vi "SaveConfig_AxisSpace.vi"(8 "error in (no error)":errorcluster, 10 "Axis Space Config":T1 {"Axis" items=["Axis 1"=1, "Axis 2"=2, "Axis 3"=3, "Axis 4"=4, "Axis 5"=5, "Axis 6"=6, "Axis 7"=7, "Axis 8"=8]}, 11 "Path (.AxisSpace.cfg)":path) -> (0 "error out":errorcluster)   [LabVIEW 2010]
doc: "Save axis space configuration to XML file."
uses:
  Typedefs/AxisSpaceCfg_ArrayofAxisCfg.ctl
  Typedefs/AxisCfg_cluster.ctl
  <vilib>/Motion/FlexMotion/CustomControls/CustomControls.llb/Axis To Read.flx
  <vilib>/Utility/xml.llb/Write to XML File(string).vi
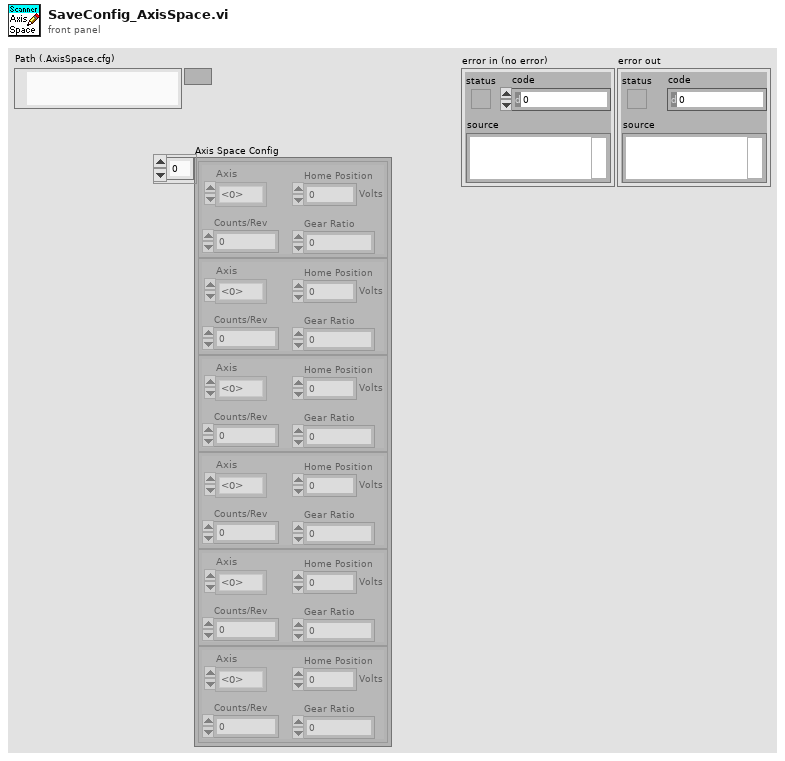
[diagram p1: front panel]
types:
  T1 = typedef "AxisSpaceCfg_ArrayofAxisCfg.ctl" = T2[]
  T2 = typedef "AxisCfg_cluster.ctl" = cluster{"Axis":T3, "Counts/Rev":dbl, "Gear Ratio":dbl, "Home Position":dbl}
  T3 = typedef "Axis To Read.flx" = u16
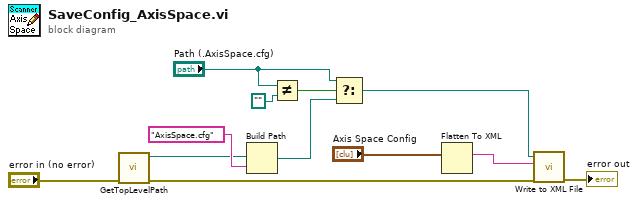
[diagram p0: block diagram]
diagram:
  n1 = call "GetTopLevelPath.vi"("error in"="error in (no error)") -> ("error out"=w2:errorcluster, "path"=w4:path)  [unwired: 9 in]
  n2 = Build Path(base path=w4, name or relative path="AxisSpace.cfg" ("file name")) -> (appended path=w8:path)
  n3 = Not Equal?(x="Path (.AxisSpace.cfg)", y=path "") -> (x != y?=w10:bool)
  n4 = Select(t="Path (.AxisSpace.cfg)", s=w10, f=w8) -> (s? t:f=w5:path)
  n5 = Flatten To XML(anything="Axis Space Config") -> (xml string=w7:string)
  n6 = call-poly <vilib>:"Write to XML File.vi"("error in (no error)"=w2, "XML Input"=w7, "XML File Path"=w5) -> ("error out"=→"error out":errorcluster)  [unwired: 6 in, 2 out]
